vi "Stby bei Pause.vi"(11 "ausgewählte Funktion":T1) -> ()   [LabVIEW 2020, in "ABB-EL3000.lvlib" / "FID.lvlib"]
uses:
  FID.lvlib
  Funktionstasten/Zustaende.ctl
  Status Analysatoren/Aktion Status Analysatoren.ctl
  Aktion STY_MES.ctl
  Status Analysatoren/Status Analysatoren.lvlib
  Funktionstasten/Funktionstasten.lvlib
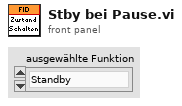
[diagram p1: front panel]
types:
  T1 = typedef "Funktionstasten.lvlib/Zustaende.ctl" = enum16{"Standby", "Pause", "Eco", "Messen", "Kalibrieren", "Spülen Filter", "Spülen Leitung", "Umgebungsluft", "0-Gas", "Cal-Gas", "CG zu PNS", "-------------", "Init 1", "Init 2", "Init 3", "Init 4", "Messen vorbereiten", "Messen durchführen", "Exit"}
  T2 = typedef "Status Analysatoren.lvlib/Aktion Status Analysatoren.ctl" = enum16{"lesen", "initialisieren", "Analysatoren aktiv", "FTIR Fehler", "FID Fehler", "PMA Fehler", "Felder einfärben"}
  T3 = typedef "Aktion STY_MES.ctl" = enum16{"lesen", "setze STY", "setze MES", "MODBUS schreiben"}
  T4 = typedef "Status Analysatoren.lvlib/Status.ctl" = cluster{"FT-IR aktiv":bool, "FT-IR Fehler":bool, "FID aktiv":bool, "FID Fehler":bool, "PMA aktiv":bool, "PMA Fehler":bool}
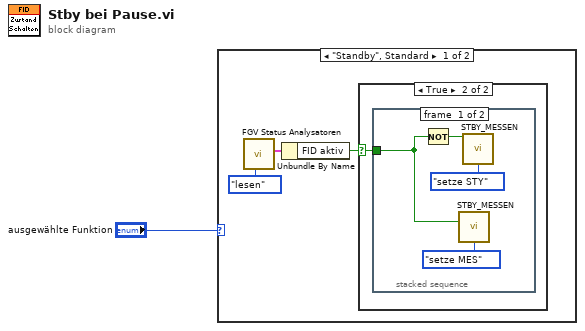
[diagram p0: block diagram]
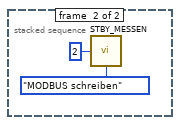
[diagram p3: hidden frame]
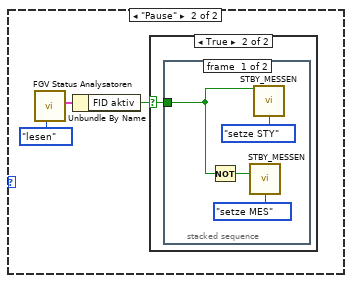
[diagram p4: hidden frame]
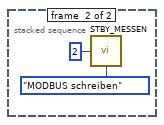
[diagram p6: hidden frame]
diagram:
  n1 = case shown="\"Standby\", Standard" "ausgewählte Funktion" {
    frame "Standby", Default {
      n2 = call "FGV Status Analysatoren.vi"("Aktionen"=Aktion_Status_Analysatoren."lesen") -> ("Status Analysatoren"=w3:T4)  [unwired: 10 in]
      n3 = Unbundle By Name(w3) -> ("FID aktiv"=w2:bool)
      n4 = case shown="True" w2 {
        selector: w2 -> [_ w5]
        frame False {
        }
        frame True {
          n5 = stacked-sequence {
            tunnel: w5 -> [w6 _]
            frame #0 {
              n6 = Not(x=w6) -> (.not. x?=w7:bool)
              n7 = call "STBY_MESSEN.vi"("Messen"=w6, "Aktion"=Aktion_STY_MES."setze MES") -> ()  [unwired: 10 in, 4 out]
              n8 = call "STBY_MESSEN.vi"("Standby"=w7, "Aktion"=Aktion_STY_MES."setze STY") -> ()  [unwired: 10 in, 4 out]
            }
            frame #1 {
              n9 = call "STBY_MESSEN.vi"("Case Nr."=2, "Aktion"=Aktion_STY_MES."MODBUS schreiben") -> ()  [unwired: 10 in, 4 out]
            }
          }
        }
      }
    }
    frame "Pause" {
      n10 = call "FGV Status Analysatoren.vi"("Aktionen"=Aktion_Status_Analysatoren."lesen") -> ("Status Analysatoren"=w13:T4)  [unwired: 10 in]
      n11 = Unbundle By Name(w13) -> ("FID aktiv"=w12:bool)
      n12 = case shown="True" w12 {
        selector: w12 -> [_ w15]
        frame False {
        }
        frame True {
          n13 = stacked-sequence {
            tunnel: w15 -> [w16 _]
            frame #0 {
              n14 = Not(x=w16) -> (.not. x?=w17:bool)
              n15 = call "STBY_MESSEN.vi"("Messen"=w17, "Aktion"=Aktion_STY_MES."setze MES") -> ()  [unwired: 10 in, 4 out]
              n16 = call "STBY_MESSEN.vi"("Standby"=w16, "Aktion"=Aktion_STY_MES."setze STY") -> ()  [unwired: 10 in, 4 out]
            }
            frame #1 {
              n17 = call "STBY_MESSEN.vi"("Case Nr."=2, "Aktion"=Aktion_STY_MES."MODBUS schreiben") -> ()  [unwired: 10 in, 4 out]
            }
          }
        }
      }
    }
  }
